vi "Write Type Override.vi"(8 "error in (no error)":errorcluster, 10 "Type Override":string, 11 "CIF_Fifo_Raw_Multi in":refnum<class "CIF_Fifo_Raw_Multi.lvclass">) -> (0 "error out":errorcluster, 3 "CIF_Fifo_Raw_Multi out":refnum<class "CIF_Fifo_Raw_Multi.lvclass">)   [LabVIEW 2021, in "CIF_Fifo_Raw_Multi.lvclass"]
uses:
  CIF_Fifo_Raw_Multi.lvclass
  CIF_Fifo_Raw_Multi.lvclass/CIF_Fifo_Raw_Multi.ctl
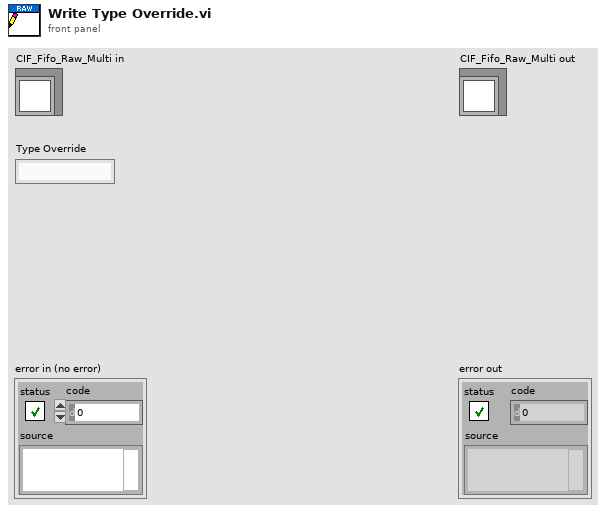
[diagram p1: front panel]
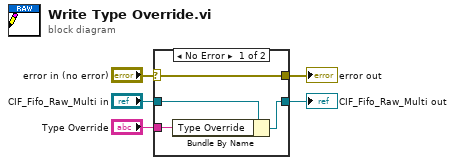
[diagram p0: block diagram]
diagram:
  n1 = case shown="No Error" "error in (no error)" {
    selector: "error in (no error)" -> [w9 w10]
    tunnel: [w9 w10] -> w4
    tunnel: [w7 w11] -> w2
    tunnel: "CIF_Fifo_Raw_Multi in" -> [w8 w11]
    tunnel: "Type Override" -> [w6 _]
    frame No Error {
      n2 = Bundle By Name(cluster=w8, "Type Override"=w6) -> (w7:refnum<class "CIF_Fifo_Raw_Multi.lvclass">)
    }
    frame Error {
    }
  }
  "error out" <- w4
  "CIF_Fifo_Raw_Multi out" <- w2
